vi "BRig_dataCurrent_Cue2_I_1A_Sel.vi"() -> (2 "output_Cue2_I_1A_Sel":i32)   [LabVIEW 2014]
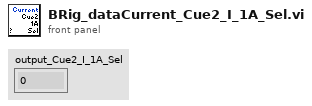
[diagram p1: front panel]
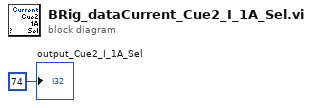
[diagram p0: block diagram]
diagram:
  "output_Cue2_I_1A_Sel" <- 74 ("output_iBlock")
